vi "Receive.vi"(6 "Timeout":T1={"mode"=enum."Relative", "deadline (ms)"=30000}, 8 "error in (no error)":errorcluster, 9 "request id":u32, 10 "session in":refnum<class "Session.lvclass">, 11 "NI_SFTP.lvlib:hardlink_openssh.com.lvclass":refnum<class "hardlink_openssh.com.lvclass">) -> (0 "error out":errorcluster, 1 "unused":i32, 2 "session out":refnum<class "Session.lvclass">, 3 "NI_SFTP.lvlib:hardlink_openssh.com.lvclass 2":refnum<class "hardlink_openssh.com.lvclass">)   [LabVIEW 2020, in "NI_SFTP.lvlib" / "hardlink_openssh.com.lvclass"]
uses:
  <vilib>/net/SFTP/API/Support/Command/hardlink_openssh.com/hardlink_openssh.com.lvclass
  <vilib>/net/SFTP/Session/Session.lvclass
  <vilib>/Utility/Deadline/Deadline.ctl
  <vilib>/Utility/Deadline/Mode.ctl
  <vilib>/net/SFTP/API/Support/Command/SSH_FXP_EXTENDED/SSH_FXP_EXTENDED.lvclass
  <vilib>/net/SFTP/Low Level Connection/Low Level Connection.lvclass
  <vilib>/Utility/Deadline/NI_Deadline.lvlib
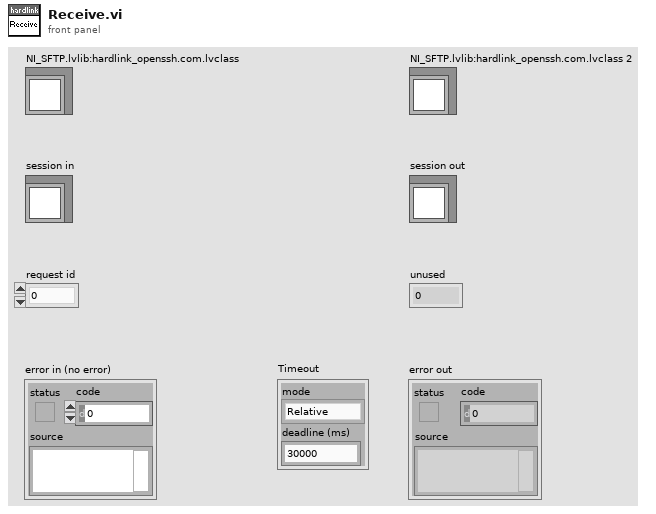
[diagram p1: front panel]
types:
  T1 = typedef "NI_Deadline.lvlib/Deadline.ctl" = cluster{"mode":T2, "deadline (ms)":u32}
  T2 = typedef "NI_Deadline.lvlib/Mode.ctl" = enum16{"Relative", "Use deadline", "Wait forever", "Nonblocking", "N/A"}
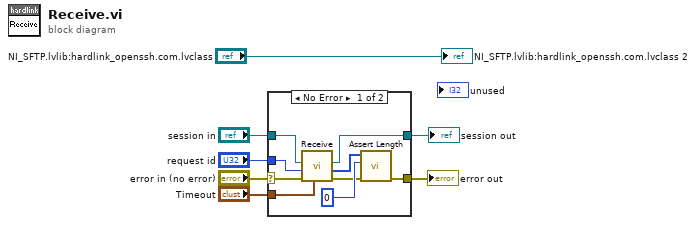
[diagram p0: block diagram]
diagram:
  n1 = case shown="No Error" "error in (no error)" {
    selector: "error in (no error)" -> [w16 w18]
    tunnel: "request id" -> [w11 _]
    tunnel: "session in" -> [w10 w17]
    tunnel: [w9 w17] -> w1
    tunnel: [w12 w18] -> w5
    tunnel: "Timeout" -> [w15 _]
    frame No Error {
      n2 = call <vilib>:"Receive.vi"("deadline"=w15, "error in (no error)"=w16, "request id"=w11, "session in"=w10) -> ("error out"=w13:errorcluster, "payload"=w8:u8[], "session out"=w9:refnum<class "Session.lvclass">)  [unwired: 4 in, 1 out]
      n3 = call <vilib>:"Assert Length.vi"("error in"=w13, "asserted length"=u32 0, "string in"=w8) -> ("error out"=w12:errorcluster)  [unwired: 7 in, 1 out]
    }
    frame Error {
    }
  }
  "error out" <- w5
  "session out" <- w1
  "NI_SFTP.lvlib:hardlink_openssh.com.lvclass 2" <- "NI_SFTP.lvlib:hardlink_openssh.com.lvclass"
